vi "Double2Config.vi"(9 "error in (no error)":errorcluster, 10 "Data":dbl, 11 "Config Address":T1 items=["ID", "Mode", "Baudrate", "Homing Offset", "Id P gain", "Id I gain", "Id D gain", "Iq P gain", "Iq I gain", "Iq D gain", "Velo P gain", "Velo I gain", "Velo D gain", "Posi P gain", "Posi I gain", "Posi D gain", "DirectForce P", "DirectForce I", "DirectForce D", "Limit Acc Max", "Limit Iq Max", "Limit Velo Max", "Limit Posi Min", "Limit Posi Max", "Voltage Min", "Voltage Max", "Watchdog", "Temperature Low", "Temperature High"]) -> (1 "error out":errorcluster, 3 "data string":string)   [LabVIEW 2016, in "GEN_2.lvlib"]
uses:
  GEN_2.lvlib
  GEN2_Config_Addr.ctl
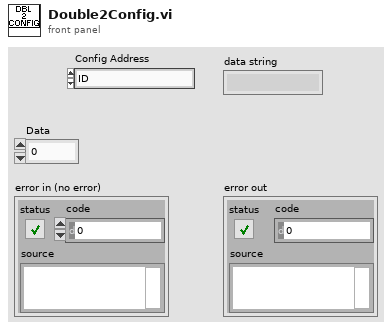
[diagram p1: front panel]
types:
  T1 = typedef "GEN_2.lvlib/GEN2_Config_Addr.ctl" = u8
  T2 = enum16{"big-endian, network order", "native, host order", "little-endian"}
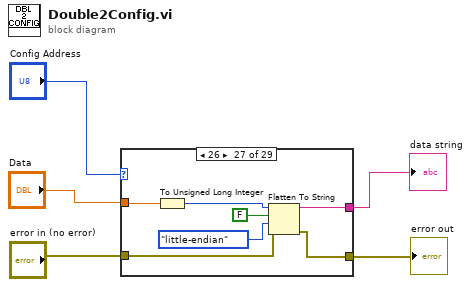
[diagram p0: block diagram]
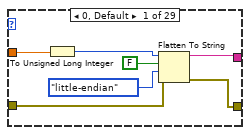
[diagram p2: hidden frame]
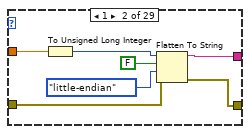
[diagram p3: hidden frame]
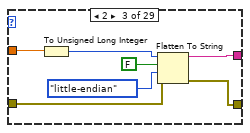
[diagram p4: hidden frame]
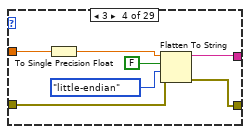
[diagram p5: hidden frame]
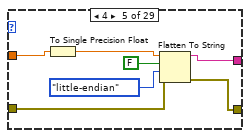
[diagram p6: hidden frame]
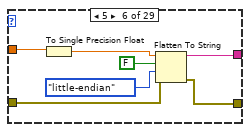
[diagram p7: hidden frame]
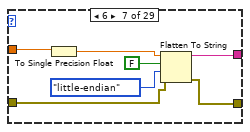
[diagram p8: hidden frame]
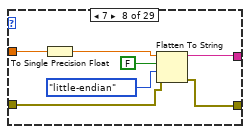
[diagram p9: hidden frame]
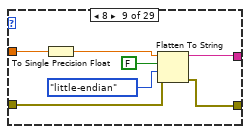
[diagram p10: hidden frame]
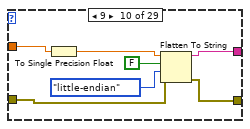
[diagram p11: hidden frame]
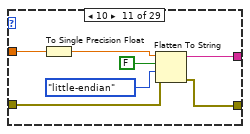
[diagram p12: hidden frame]
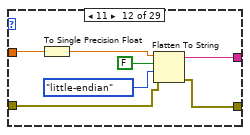
[diagram p13: hidden frame]
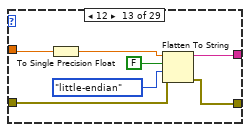
[diagram p14: hidden frame]
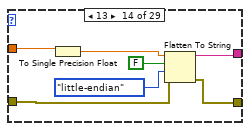
[diagram p15: hidden frame]
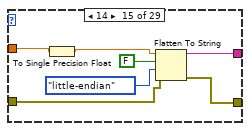
[diagram p16: hidden frame]
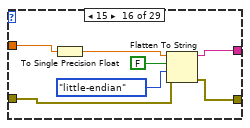
[diagram p17: hidden frame]
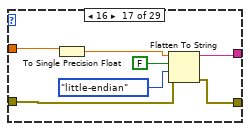
[diagram p18: hidden frame]
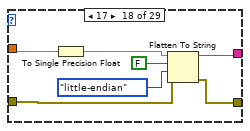
[diagram p19: hidden frame]
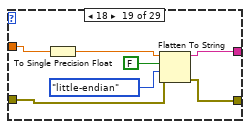
[diagram p20: hidden frame]
diagram:
  n1 = case shown="26" "Config Address" {
    tunnel: [w9 w19 w24 w29 w36 w44 w51 w58 w62 w69 w76 w86 w90 w100 w108 w111 w121 w125 w135 w139 w149 w153 w163 w170 w174 w184 w188 w198 w205] -> w2
    tunnel: "Data" -> [w8 w15 w21 w30 w34 w41 w48 w55 w65 w72 w79 w83 w93 w97 w105 w114 w118 w128 w132 w142 w146 w156 w160 w167 w177 w181 w191 w195 w202]
    tunnel: [w6 w14 w23 w28 w37 w43 w50 w57 w63 w70 w77 w85 w91 w99 w107 w112 w120 w126 w134 w140 w148 w154 w162 w169 w175 w183 w189 w197 w204] -> w5
    tunnel: "error in (no error)" -> [w7 w13 w22 w27 w35 w42 w49 w56 w64 w71 w78 w84 w92 w98 w106 w113 w119 w127 w133 w141 w147 w155 w161 w168 w176 w182 w190 w196 w203]
    frame 0, Default {
      n2 = To Unsigned Long Integer(number=w8) -> (unsigned 32bit integer=w12:u32)
      n3 = Flatten To String(anything=w12, prepend array or string size? (T)=FALSE, byte order (0:big-endian, network order)=T2."little-endian", error in (no error)=w7) -> (data string=w9:string, error out=w6:errorcluster)  [unwired: 1 out]
    }
    frame 1 {
      n4 = To Unsigned Long Integer(number=w15) -> (unsigned 32bit integer=w16:u32)
      n5 = Flatten To String(anything=w16, prepend array or string size? (T)=FALSE, byte order (0:big-endian, network order)=T2."little-endian", error in (no error)=w13) -> (data string=w19:string, error out=w14:errorcluster)  [unwired: 1 out]
    }
    frame 2 {
      n6 = To Unsigned Long Integer(number=w21) -> (unsigned 32bit integer=w20:u32)
      n7 = Flatten To String(anything=w20, prepend array or string size? (T)=FALSE, byte order (0:big-endian, network order)=T2."little-endian", error in (no error)=w22) -> (data string=w24:string, error out=w23:errorcluster)  [unwired: 1 out]
    }
    frame 3 {
      n8 = To Single Precision Float(number=w30) -> (single precision float=w31:sgl)
      n9 = Flatten To String(anything=w31, prepend array or string size? (T)=FALSE, byte order (0:big-endian, network order)=T2."little-endian", error in (no error)=w27) -> (data string=w29:string, error out=w28:errorcluster)  [unwired: 1 out]
    }
    frame 4 {
      n10 = To Single Precision Float(number=w34) -> (single precision float=w40:sgl)
      n11 = Flatten To String(anything=w40, prepend array or string size? (T)=FALSE, byte order (0:big-endian, network order)=T2."little-endian", error in (no error)=w35) -> (data string=w36:string, error out=w37:errorcluster)  [unwired: 1 out]
    }
    frame 5 {
      n12 = To Single Precision Float(number=w41) -> (single precision float=w45:sgl)
      n13 = Flatten To String(anything=w45, prepend array or string size? (T)=FALSE, byte order (0:big-endian, network order)=T2."little-endian", error in (no error)=w42) -> (data string=w44:string, error out=w43:errorcluster)  [unwired: 1 out]
    }
    frame 6 {
      n14 = To Single Precision Float(number=w48) -> (single precision float=w52:sgl)
      n15 = Flatten To String(anything=w52, prepend array or string size? (T)=FALSE, byte order (0:big-endian, network order)=T2."little-endian", error in (no error)=w49) -> (data string=w51:string, error out=w50:errorcluster)  [unwired: 1 out]
    }
    frame 7 {
      n16 = To Single Precision Float(number=w55) -> (single precision float=w59:sgl)
      n17 = Flatten To String(anything=w59, prepend array or string size? (T)=FALSE, byte order (0:big-endian, network order)=T2."little-endian", error in (no error)=w56) -> (data string=w58:string, error out=w57:errorcluster)  [unwired: 1 out]
    }
    frame 8 {
      n18 = To Single Precision Float(number=w65) -> (single precision float=w66:sgl)
      n19 = Flatten To String(anything=w66, prepend array or string size? (T)=FALSE, byte order (0:big-endian, network order)=T2."little-endian", error in (no error)=w64) -> (data string=w62:string, error out=w63:errorcluster)  [unwired: 1 out]
    }
    frame 9 {
      n20 = To Single Precision Float(number=w72) -> (single precision float=w73:sgl)
      n21 = Flatten To String(anything=w73, prepend array or string size? (T)=FALSE, byte order (0:big-endian, network order)=T2."little-endian", error in (no error)=w71) -> (data string=w69:string, error out=w70:errorcluster)  [unwired: 1 out]
    }
    frame 10 {
      n22 = To Single Precision Float(number=w79) -> (single precision float=w80:sgl)
      n23 = Flatten To String(anything=w80, prepend array or string size? (T)=FALSE, byte order (0:big-endian, network order)=T2."little-endian", error in (no error)=w78) -> (data string=w76:string, error out=w77:errorcluster)  [unwired: 1 out]
    }
    frame 11 {
      n24 = To Single Precision Float(number=w83) -> (single precision float=w87:sgl)
      n25 = Flatten To String(anything=w87, prepend array or string size? (T)=FALSE, byte order (0:big-endian, network order)=T2."little-endian", error in (no error)=w84) -> (data string=w86:string, error out=w85:errorcluster)  [unwired: 1 out]
    }
    frame 12 {
      n26 = To Single Precision Float(number=w93) -> (single precision float=w94:sgl)
      n27 = Flatten To String(anything=w94, prepend array or string size? (T)=FALSE, byte order (0:big-endian, network order)=T2."little-endian", error in (no error)=w92) -> (data string=w90:string, error out=w91:errorcluster)  [unwired: 1 out]
    }
    frame 13 {
      n28 = To Single Precision Float(number=w97) -> (single precision float=w101:sgl)
      n29 = Flatten To String(anything=w101, prepend array or string size? (T)=FALSE, byte order (0:big-endian, network order)=T2."little-endian", error in (no error)=w98) -> (data string=w100:string, error out=w99:errorcluster)  [unwired: 1 out]
    }
    frame 14 {
      n30 = To Single Precision Float(number=w105) -> (single precision float=w104:sgl)
      n31 = Flatten To String(anything=w104, prepend array or string size? (T)=FALSE, byte order (0:big-endian, network order)=T2."little-endian", error in (no error)=w106) -> (data string=w108:string, error out=w107:errorcluster)  [unwired: 1 out]
    }
    frame 15 {
      n32 = To Single Precision Float(number=w114) -> (single precision float=w115:sgl)
      n33 = Flatten To String(anything=w115, prepend array or string size? (T)=FALSE, byte order (0:big-endian, network order)=T2."little-endian", error in (no error)=w113) -> (data string=w111:string, error out=w112:errorcluster)  [unwired: 1 out]
    }
    frame 16 {
      n34 = To Single Precision Float(number=w118) -> (single precision float=w122:sgl)
      n35 = Flatten To String(anything=w122, prepend array or string size? (T)=FALSE, byte order (0:big-endian, network order)=T2."little-endian", error in (no error)=w119) -> (data string=w121:string, error out=w120:errorcluster)  [unwired: 1 out]
    }
    frame 17 {
      n36 = To Single Precision Float(number=w128) -> (single precision float=w131:sgl)
      n37 = Flatten To String(anything=w131, prepend array or string size? (T)=FALSE, byte order (0:big-endian, network order)=T2."little-endian", error in (no error)=w127) -> (data string=w125:string, error out=w126:errorcluster)  [unwired: 1 out]
    }
    frame 18 {
      n38 = To Single Precision Float(number=w132) -> (single precision float=w136:sgl)
      n39 = Flatten To String(anything=w136, prepend array or string size? (T)=FALSE, byte order (0:big-endian, network order)=T2."little-endian", error in (no error)=w133) -> (data string=w135:string, error out=w134:errorcluster)  [unwired: 1 out]
    }
    frame 19 {
      n40 = To Single Precision Float(number=w142) -> (single precision float=w143:sgl)
      n41 = Flatten To String(anything=w143, prepend array or string size? (T)=FALSE, byte order (0:big-endian, network order)=T2."little-endian", error in (no error)=w141) -> (data string=w139:string, error out=w140:errorcluster)  [unwired: 1 out]
    }
    frame 20 {
      n42 = To Single Precision Float(number=w146) -> (single precision float=w150:sgl)
      n43 = Flatten To String(anything=w150, prepend array or string size? (T)=FALSE, byte order (0:big-endian, network order)=T2."little-endian", error in (no error)=w147) -> (data string=w149:string, error out=w148:errorcluster)  [unwired: 1 out]
    }
    frame 21 {
      n44 = To Single Precision Float(number=w156) -> (single precision float=w157:sgl)
      n45 = Flatten To String(anything=w157, prepend array or string size? (T)=FALSE, byte order (0:big-endian, network order)=T2."little-endian", error in (no error)=w155) -> (data string=w153:string, error out=w154:errorcluster)  [unwired: 1 out]
    }
    frame 22 {
      n46 = To Single Precision Float(number=w160) -> (single precision float=w164:sgl)
      n47 = Flatten To String(anything=w164, prepend array or string size? (T)=FALSE, byte order (0:big-endian, network order)=T2."little-endian", error in (no error)=w161) -> (data string=w163:string, error out=w162:errorcluster)  [unwired: 1 out]
    }
    frame 23 {
      n48 = To Single Precision Float(number=w167) -> (single precision float=w171:sgl)
      n49 = Flatten To String(anything=w171, prepend array or string size? (T)=FALSE, byte order (0:big-endian, network order)=T2."little-endian", error in (no error)=w168) -> (data string=w170:string, error out=w169:errorcluster)  [unwired: 1 out]
    }
    frame 24 {
      n50 = To Single Precision Float(number=w177) -> (single precision float=w178:sgl)
      n51 = Flatten To String(anything=w178, prepend array or string size? (T)=FALSE, byte order (0:big-endian, network order)=T2."little-endian", error in (no error)=w176) -> (data string=w174:string, error out=w175:errorcluster)  [unwired: 1 out]
    }
    frame 25 {
      n52 = To Single Precision Float(number=w181) -> (single precision float=w185:sgl)
      n53 = Flatten To String(anything=w185, prepend array or string size? (T)=FALSE, byte order (0:big-endian, network order)=T2."little-endian", error in (no error)=w182) -> (data string=w184:string, error out=w183:errorcluster)  [unwired: 1 out]
    }
    frame 26 {
      n54 = To Unsigned Long Integer(number=w191) -> (unsigned 32bit integer=w192:u32)
      n55 = Flatten To String(anything=w192, prepend array or string size? (T)=FALSE, byte order (0:big-endian, network order)=T2."little-endian", error in (no error)=w190) -> (data string=w188:string, error out=w189:errorcluster)  [unwired: 1 out]
    }
    frame 27 {
      n56 = To Single Precision Float(number=w195) -> (single precision float=w199:sgl)
      n57 = Flatten To String(anything=w199, prepend array or string size? (T)=FALSE, byte order (0:big-endian, network order)=T2."little-endian", error in (no error)=w196) -> (data string=w198:string, error out=w197:errorcluster)  [unwired: 1 out]
    }
    frame 28 {
      n58 = To Single Precision Float(number=w202) -> (single precision float=w206:sgl)
      n59 = Flatten To String(anything=w206, prepend array or string size? (T)=FALSE, byte order (0:big-endian, network order)=T2."little-endian", error in (no error)=w203) -> (data string=w205:string, error out=w204:errorcluster)  [unwired: 1 out]
    }
  }
  "error out" <- w5
  "data string" <- w2
